vi "Agilent 34970 Setup Temperature HEWH.vi"(6 "LV Program":T1, 8 "Error In":errorcluster, 10 "Agilent Channel Input":string="111,112,113,114,115,116,109,110,201,202,203,204,205,206,207,208,209,210,211,212,213,214,215,216,107,108,301,302,303,304,305,306,307,308,309,310,311,312,313,314,315,316,105,106", 11 "VISA Refnum in":refnum<visa-resource-name>) -> (0 "Error Out":errorcluster, 3 "VISA Resource Name Out":refnum<visa-resource-name>)   [LabVIEW 2020]
uses:
  Trunk/Utility/Save File/File Setup (Public)/Type Definition/Save File DOE LabView Program.ctl
  Agilent 34970.lvlib
  Trunk/Utility/Save File/File Setup.lvlib
panel:
  in  "DEBUG":string="111,112,113,114,115,116,109,110,201,202,203,204,205,206,207,208,209,210,211,212,213,214,215,216,107,108,301,302,303,304,305,306,307,308,309,310,311,312,313,314,315,316,105,106"
  # "111,112,113,114,115,116,109,110,201,202,203,204,205,206,207,208,209,210,211,212,213,214,215,216,107,108,301,302,303,304,305,306,307,308,309,310,311,312,313,314,315,316,105,106"
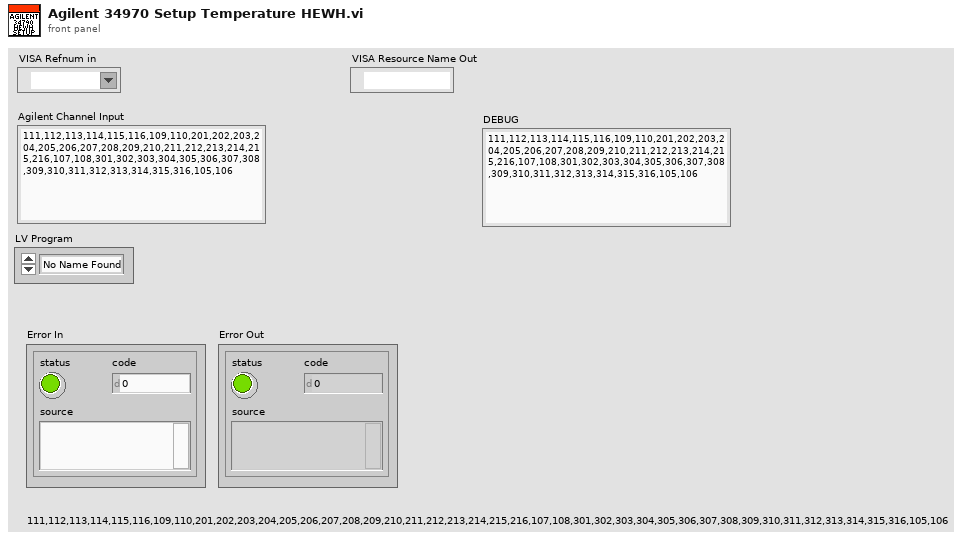
[diagram p1: front panel]
types:
  T1 = typedef "File Setup.lvlib/Save File DOE LabView Program.ctl" = enum16{"No Name Found", "DOE Stand", "Dishwasher Kitchen", "Portable Stand", "HEWH", "Dryer", "Dryer WILT", "HCC", "PRAT", "HEWH RLT", "Refrigeration", "Gas Water Heater"}
  T2 = cluster{"Thermocouple Type (Last)":enum16{"B", "E", "J", "K", "N", "R", "S", "T", "Default (Last)"}, "TC Rjunction (2:Int)":enum16{"Fixed", "External", "Internal"}, "Fixed Rjunction Temp (0:Manual)":enum16{"Manual", "Minimum", "Maximum"}, "TC Auto Check? (F:Don't Check)":bool, "Rjunct Temp Value (0)":dbl}
  T3 = enum16{"Thermocouple", "Thermistor", "RTD", "4-Wire RTD"}
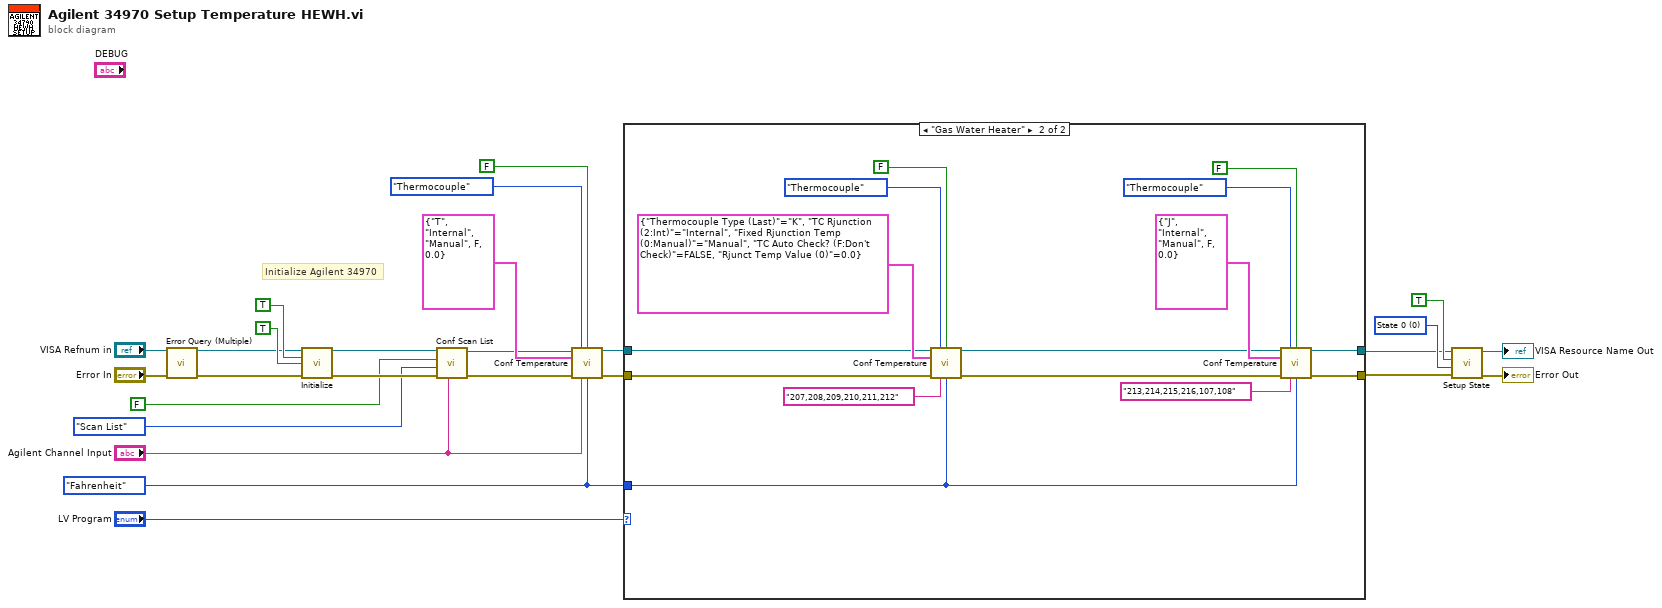
[diagram p0: block diagram]
diagram:
  w5 = u16 0 items=["State 0", "State 1", "State 2", "State 3", "State 4", "State 5", "Preset State"] ("Setup State (6:Preset)")
  w9 = enum16{"Celsius", "Fahrenheit", "Kelvin"}."Fahrenheit" ("Units (0:Celsius)")
  # "Initialize Agilent 34970"
  n1 = call "Error Query (Multiple).vi"("VISA Resource Name"="VISA Refnum in", "error in (no error)"="Error In") -> ("VISA Resource Name Out"=w20:refnum<visa-resource-name>, "error out"=w21:errorcluster)  [unwired: 10 in, 2 out]
  n2 = call "Initialize.vi"("VISA Resource Name"=w20, "ID Query (T: Check)"=TRUE, "Reset (T: Reset)"=TRUE, "error in (no error)"=w21) -> ("VISA Resource Name Out"=w25:refnum<visa-resource-name>, "error out"=w26:errorcluster)  [unwired: 10 in]
  n3 = call "Conf Scan List.vi"("Scan List (empty)"="Agilent Channel Input", "error in (no error)"=w26, "Check Parameter (0:Scan List)"=enum16{"Scan List", "Scan Size"}."Scan List", "Set/Check (F:Set)"=FALSE, "VISA Resource Name"=w25) -> ("error out"=w15:errorcluster, "VISA Resource Name Out"=w16:refnum<visa-resource-name>)  [unwired: 4 in, 1 out]
  n4 = call "Conf Temperature.vi"("VISA Resource Name"=w16, "Transducer Type (0:TC)"=T3."Thermocouple", "Set/Check? (F:Set)"=FALSE, "Thermocouple Configuration"=T2 {"Thermocouple Type (Last)"=enum."T", "TC Rjunction (2:Int)"=enum."Internal", "Fixed Rjunction Temp (0:Manual)"=enum."Manual", "TC Auto Check? (F:Don't Check)"=FALSE, "Rjunct Temp Value (0)"=0.0}, "error in (no error)"=w15, "Channel List(empty)"="Agilent Channel Input", "Units (0:Celsius)"=w9) -> ("VISA Resource Name Out"=w10:refnum<visa-resource-name>, "error out"=w12:errorcluster)  [unwired: 6 in, 1 out]
  n5 = case shown="\"Gas Water Heater\"" "LV Program" {
    tunnel: w12 -> [w28 w34]
    tunnel: [w28 w35] -> w4
    tunnel: w10 -> [w27 w33]
    tunnel: w9 -> [_ w30]
    tunnel: [w27 w29] -> w3
    frame Default {
    }
    frame "Gas Water Heater" {
      n6 = call "Conf Temperature.vi"("VISA Resource Name"=w33, "Transducer Type (0:TC)"=T3."Thermocouple", "Set/Check? (F:Set)"=FALSE, "Thermocouple Configuration"=T2 {"Thermocouple Type (Last)"=enum."K", "TC Rjunction (2:Int)"=enum."Internal", "Fixed Rjunction Temp (0:Manual)"=enum."Manual", "TC Auto Check? (F:Don't Check)"=FALSE, "Rjunct Temp Value (0)"=0.0}, "error in (no error)"=w34, "Channel List(empty)"="207,208,209,210,211,212" ("Scan List (empty)"), "Units (0:Celsius)"=w30) -> ("VISA Resource Name Out"=w31:refnum<visa-resource-name>, "error out"=w32:errorcluster)  [unwired: 6 in, 1 out]
      n7 = call "Conf Temperature.vi"("VISA Resource Name"=w31, "Transducer Type (0:TC)"=T3."Thermocouple", "Set/Check? (F:Set)"=FALSE, "Thermocouple Configuration"=T2 {"Thermocouple Type (Last)"=enum."J", "TC Rjunction (2:Int)"=enum."Internal", "Fixed Rjunction Temp (0:Manual)"=enum."Manual", "TC Auto Check? (F:Don't Check)"=FALSE, "Rjunct Temp Value (0)"=0.0}, "error in (no error)"=w32, "Channel List(empty)"="213,214,215,216,107,108" ("Scan List (empty)"), "Units (0:Celsius)"=w30) -> ("VISA Resource Name Out"=w29:refnum<visa-resource-name>, "error out"=w35:errorcluster)  [unwired: 6 in, 1 out]
    }
  }
  n8 = call "Setup State.vi"("error in (no error)"=w4, "Setup State (6:Preset)"=w5, "Recall/Save (F=Recall)"=TRUE, "VISA Resource Name"=w3) -> ("error out"=→"Error Out":errorcluster, "VISA Resource Name Out"=→"VISA Resource Name Out":refnum<visa-resource-name>)  [unwired: 6 in]
